vi "mainOCR _PC.vi"() -> ()   [LabVIEW 2025]
uses:
  ocr/ocr.lvclass
  ocr/TextDecRecResult2L.ctl
  <vilib>/vision/Image Controls.llb/IMAQ Image.ctl
panel:
  out "uploadSucc":i32
  out "InitRecDec Success":string
  out "Numeric":i32
  out "Image":T1(plugin-control)
  in  "stop":bool
  in  "NEXT Button":bool
  in  "device 2":enum16{"CPU", "GPU0"}(ring)
  in  "PathImage 2":path=path "D:/Test/dllTest/images_2"
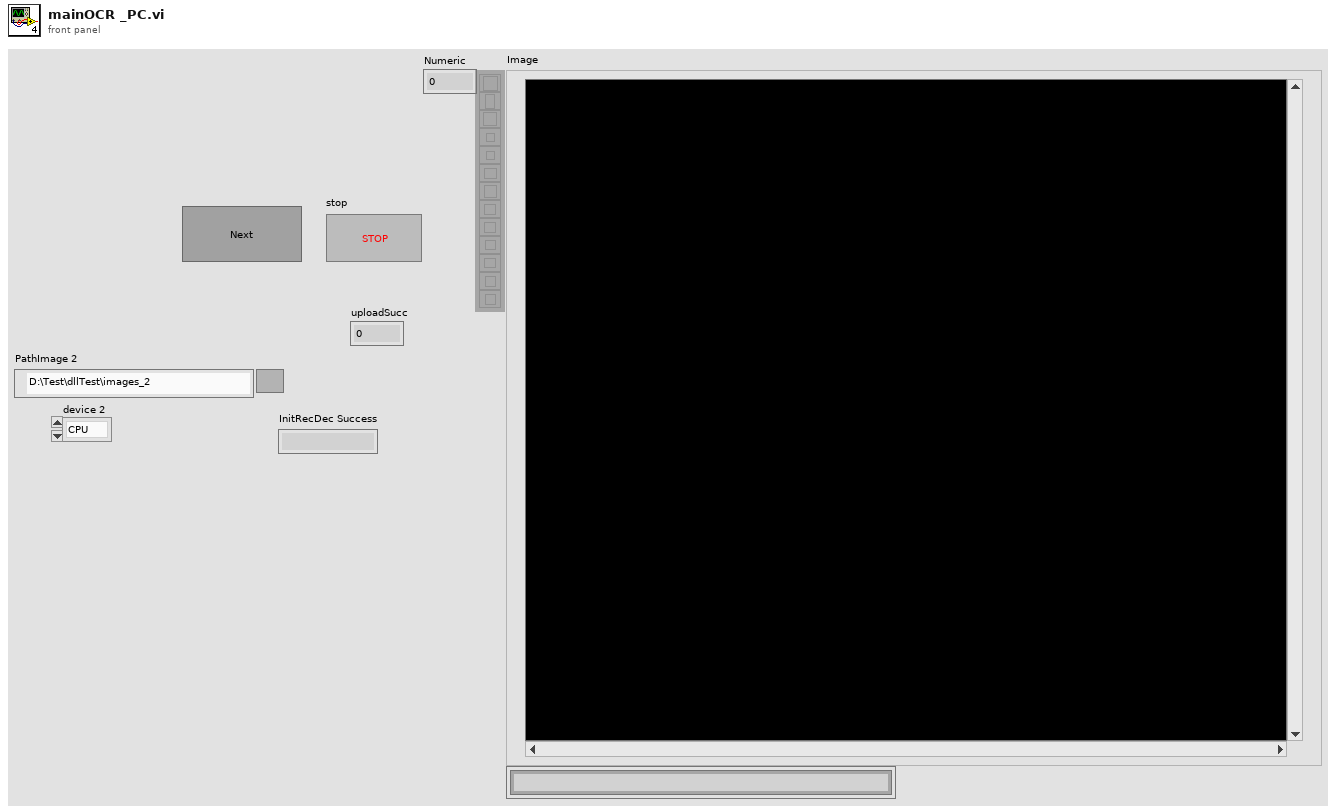
[diagram p1: front panel]
types:
  T1 = typedef "IMAQ Image.ctl" = refnum<image>
  T2 = typedef "adsOCR.lvlib/ocr.lvclass/TextDecRecResult2L.ctl" = cluster{"imgIdx":i32, "TLx":i32, "TLy":i32, "BRx":i32, "BRy":i32, "angle":sgl, "txtLen":i32}
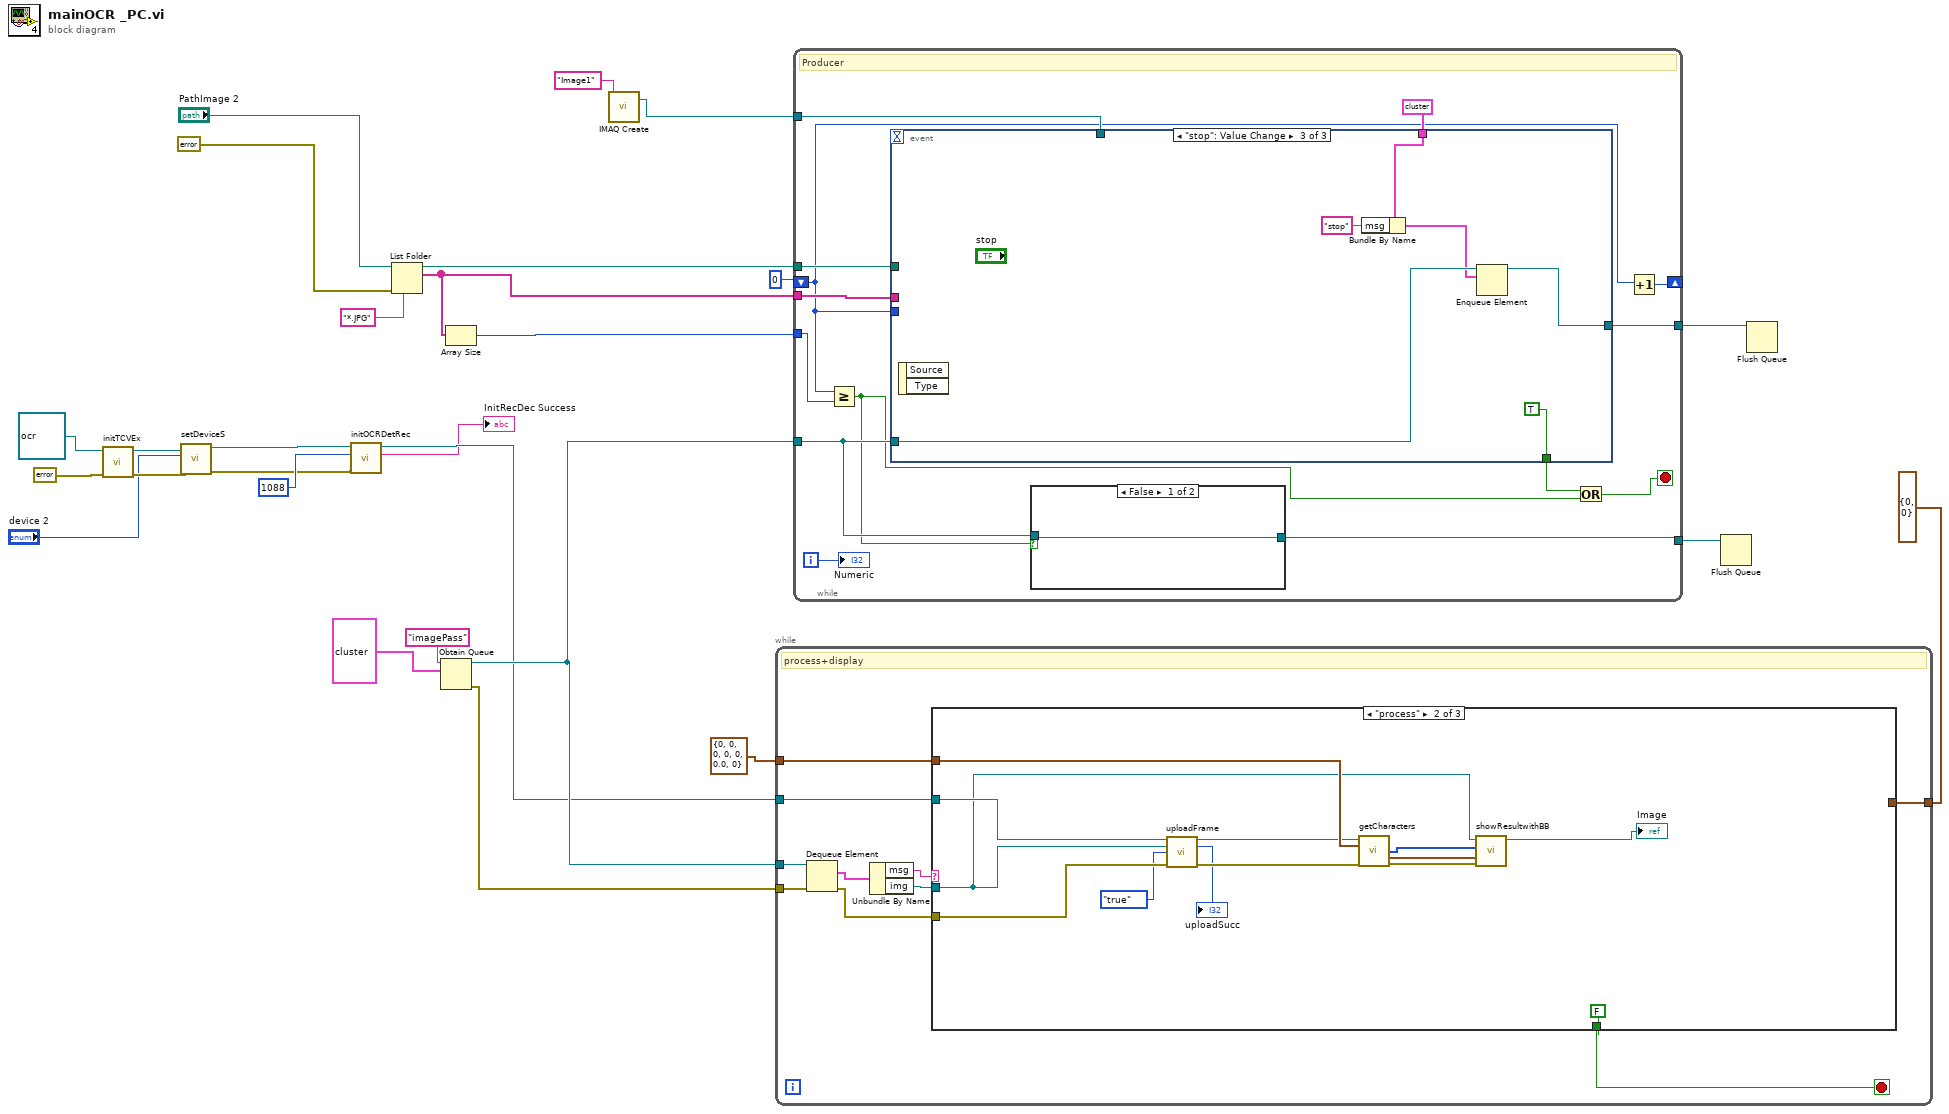
[diagram p0: block diagram]
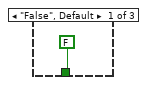
[diagram p2: hidden frame]
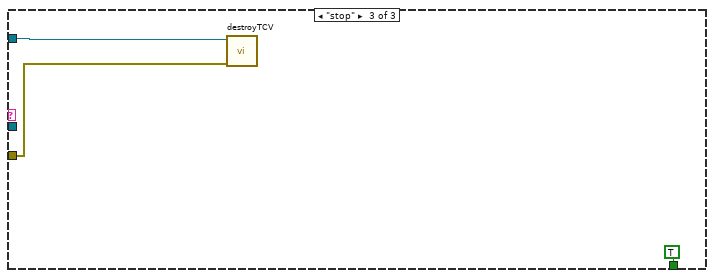
[diagram p3: hidden frame]
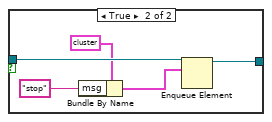
[diagram p4: hidden frame]
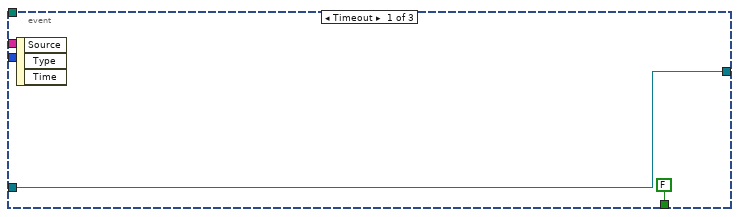
[diagram p5: hidden frame]
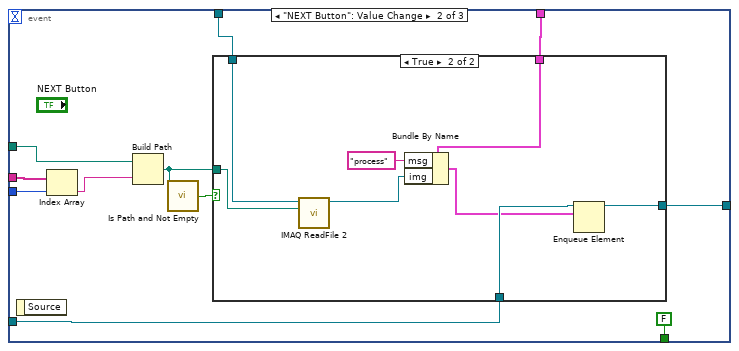
[diagram p6: hidden frame]
diagram:
  n1 = call-dynamic "initTCVEx.vi"("error in (no error)"=errorcluster {"status"=FALSE, "code"=0, "source"=""}, "ocr in"=refnum<class "ocr.lvclass"> refnum) -> ("error out"=w22:errorcluster, "ocr out"=w23:refnum<class "ocr.lvclass">)  [unwired: 8 in]
  n2 = call-dynamic "setDeviceS.vi"("error in (no error)"=w22, "devices"="device 2", "ocr in"=w23) -> ("error out"=w2:errorcluster, "ocr out"=w5:refnum<class "ocr.lvclass">)  [unwired: 6 in, 1 out]
  n3 = call-dynamic "initOCRDetRec.vi"("error in (no error)"=w2, "targetSize"=1088, "ocr in"=w5) -> ("InitRecDec Success"=→"InitRecDec Success":string, "ocr out"=w4:refnum<class "ocr.lvclass">)  [unwired: 5 in, 2 out]
  n4 = List Folder(path="PathImage 2", pattern="*.JPG", error in=errorcluster {"status"=FALSE, "code"=0, "source"=""}) -> (path out=w19:path, filenames=w11:string[])  [unwired: 1 in, 2 out]
  n5 = Obtain Queue(name (unnamed)="imagePass", element data type=cluster{"msg":string, "img":T1} {"msg"="", "img"=refnum}) -> (queue out=w12:refnum<queue>, error out=w9:errorcluster)  [unwired: 3 in, 1 out]
  n6 = Array Size(array=w11) -> (size(s)=w17:i32)
  n7 = call "IMAQ Create"("Image Name"="Image1") -> ("New Image"=w15:T1)  [unwired: 4 in, 1 out]
  n8 = while {
    tunnel: cluster{"x":i32, "y":i32} {"x"=0, "y"=0} -> [w32]
    tunnel: w12 -> [w37]
    tunnel: w4 -> [w33]
    tunnel: w9 -> [w30]
    tunnel: T2 {"imgIdx"=0, "TLx"=0, "TLy"=0, "BRx"=0, "BRy"=0, "angle"=0.0, "txtLen"=0} ("Cluster") -> [w28]
    stop <- w31 stop-if-true
    # "process+display"
    n9 = Dequeue Element(queue=w37, error in (no error)=w30) -> (element=w36:cluster{"msg":string, "img":T1}, error out=w29:errorcluster)  [unwired: 1 in, 2 out]
    n10 = Unbundle By Name(w36) -> ("msg"=w35:string, "img"=w34:T1)
    n11 = case shown="\"process\"" w35 {
      tunnel: w34 -> [_ w44 _]
      tunnel: w33 -> [_ w49 w54]
      tunnel: w32 -> [_ _ _]
      tunnel: [FALSE FALSE TRUE] -> w31
      tunnel: w29 -> [_ w47 w52]
      tunnel: w28 -> [_ w50 _]
      frame "False", Default {
      }
      frame "process" {
        n12 = call-dynamic "uploadFrame.vi"("ocr in"=w49, "Image"=w44, "normalise"=enum32{"false", "true"}."true", "error in (no error)"=w47) -> ("ocr out"=w48:refnum<class "ocr.lvclass">, "uploadSucc"=→"uploadSucc":i32, "error out"=w45:errorcluster)  [unwired: 8 in, 1 out]
        n13 = call-dynamic "getCharacters.vi"("ocr in"=w48, "Cluster"=w50, "error in (no error)"=w45) -> ("chars"=w43:u8[], "TextDecRecResult2L"=w41:T2[], "error out"=w42:errorcluster)  [unwired: 8 in, 2 out]
        n14 = call "showResultwithBB.vi"("error in"=w42, "Array"=w41, "chars"=w43, "Image in"=w44) -> ("Image out"=→"Image":T1)  [unwired: 4 in, 1 out]
      }
      frame "stop" {
        n15 = call-dynamic "destroyTCV.vi"("error in (no error)"=w52, "ocr in"=w54) -> ()  [unwired: 8 in, 2 out]
      }
    }
  }
  n16 = while {
    shift-right: [w64] -> _
    shift-left: 0 -> [w56]
    tunnel: w19 -> [w68]
    tunnel: w11 -> [w67]
    tunnel: w17 -> [w66]
    tunnel: w15 -> [w65]
    tunnel: w12 -> [w59]
    tunnel: [w60] -> w8
    tunnel: [w57] -> w7
    i -> [w55]
    stop <- w61 stop-if-true
    # "Producer"
    n17 = Greater Or Equal?(x=w56, y=w66) -> (x >= y?=w58:bool)
    n18 = event shown="[2] \"stop\": Value Change" {
      selector: _ -> [_ _ _]
      dyn-events: _ -> [_ _ _]
      timeout: _ -> [_ _ _]
      tunnel: w68 -> [_ w87 _]
      tunnel: w67 -> [_ w84 _]
      tunnel: w65 -> [_ w86 _]
      tunnel: w59 -> [w75 w85 w100]
      tunnel: w56 -> [_ w83 _]
      tunnel: cluster{"msg":string, "img":T1} {"msg"="", "img"=refnum} -> [_ w79 w102]
      tunnel: [FALSE FALSE TRUE] -> w62
      tunnel: [w75 w77 w97] -> w60
      event Timeout {
        n19 = event-data() -> ()  [unwired: 1 in, 3 out]
      }
      event "NEXT Button": Value Change {
        n20 = event-data() -> ()  [unwired: 1 in, 1 out]
        n21 = Index Array(array=w84, index=w83) -> (element=w82:string)
        n22 = Build Path(base path=w87, name or relative path=w82) -> (appended path=w81:path)
        n23 = call <vilib>:"Is Path and Not Empty.vi"("path"=w81) -> ("Is Path and Not Empty?"=w80:bool)  [unwired: 4 in]
        n24 = case shown="True" w80 {
          tunnel: w86 -> [_ w96]
          tunnel: w81 -> [_ w95]
          tunnel: w85 -> [w88 w94]
          tunnel: w79 -> [_ w90]
          tunnel: [w88 w89] -> w77
          frame False {
          }
          frame True {
            n25 = call "IMAQ ReadFile 2"("File Path"=w95, "Image"=w96) -> ("Image Out"=w92:T1)  [unwired: 5 in, 4 out]
            n26 = Bundle By Name(cluster=w90, "msg"="process", "img"=w92) -> (w91:cluster{"msg":string, "img":T1})
            n27 = Enqueue Element(queue=w94, element=w91) -> (queue out=w89:refnum<queue>)  [unwired: 2 in, 2 out]
          }
        }
      }
      event "stop": Value Change {
        n28 = event-data() -> ()  [unwired: 1 in, 2 out]
        n29 = Bundle By Name(cluster=w102, "msg"="stop") -> (w99:cluster{"msg":string, "img":T1})
        n30 = Enqueue Element(queue=w100, element=w99) -> (queue out=w97:refnum<queue>)  [unwired: 2 in, 2 out]
      }
    }
    n31 = case shown="False" w58 {
      tunnel: w59 -> [w69 w73]
      tunnel: [w69 w70] -> w57
      frame False {
      }
      frame True {
        n32 = Bundle By Name(cluster=cluster{"msg":string, "img":T1} {"msg"="", "img"=refnum}, "msg"="stop") -> (w74:cluster{"msg":string, "img":T1})
        n33 = Enqueue Element(queue=w73, element=w74) -> (queue out=w70:refnum<queue>)  [unwired: 2 in, 2 out]
      }
    }
    n34 = Or(x=w62, y=w58) -> (x .or. y?=w61:bool)
    n35 = Increment(x=w56) -> (x+1=w64:i32)
    "Numeric" <- w55
  }
  n36 = Flush Queue(queue=w7) -> ()  [unwired: 1 in, 3 out]
  n37 = Flush Queue(queue=w8) -> ()  [unwired: 1 in, 3 out]
